vi "createTestCaseXMLReport.vi"(8 "error in (no error)":errorcluster, 11 "TestTestResult.Ant":refnum<class "_TextTestResult.JUnitXML.lvclass">) -> (0 "error out":errorcluster={"status"=TRUE, "code"=1, "source"="Release Queue in _TextTestResult.Ant.lvclass:createTestCaseXMLReport.vi"}, 2 "XML Report Data":string="<testsuite disabled=\"0\" errors=\"0\" failures=\"1\" name=\"TestSuite\" tests=\"1\" time=\"3405919291.7997\"><testsuite disabled=\"0\" errors=\"0\" failures=\"2\" name=\"MixedTest TestSuite\" tests=\"3\" time=\"3405919291.7997\"><testsuite disabled=\"0\" errors=\"0\" failures=\"1\" name=\"FrameworkSubTestSuite\" tests=\"2\" time=\"1.3519439697266\"><testcase classname=\"DoNotWaitOnTestComplete\" name=\"testDemo2\" status=\"testPass\" time=\"0.010014533996582\"/><testcase classname=\"DoNotWaitOnTestComplete\" name=\"testDemo\" status=\"testFailure\" time=\"0.010014533996582\"/></TestSuite><testsuite disabled=\"0\" errors=\"0\" failures=\"2\" name=\"FrameworkSubTestSuite\" tests=\"2\" time=\"1.6123185157776\"><testcase classname=\"DoNotWaitOnTestComplete\" name=\"testDemo2\" status=\"testPass\" time=\"0.010014057159424\"/><testcase classname=\"DoNotWaitOnTestComplete\" name=\"testDemo\" status=\"testFailure\" time=\"0.010014057159424\"/><testcase classname=\"LocationOutsideClassRoot\" name=\"testOutsideRoot\" status=\"testFailure\" time=\"0.010014533996582\"/>")   [LabVIEW 2018, in "_TextTestResult.JUnitXML.lvclass"]
uses:
  _TextTestResult.JUnitXML.lvclass
  _TextTestResult.JUnitXML.lvclass/_TextTestResult.JUnitXML.ctl
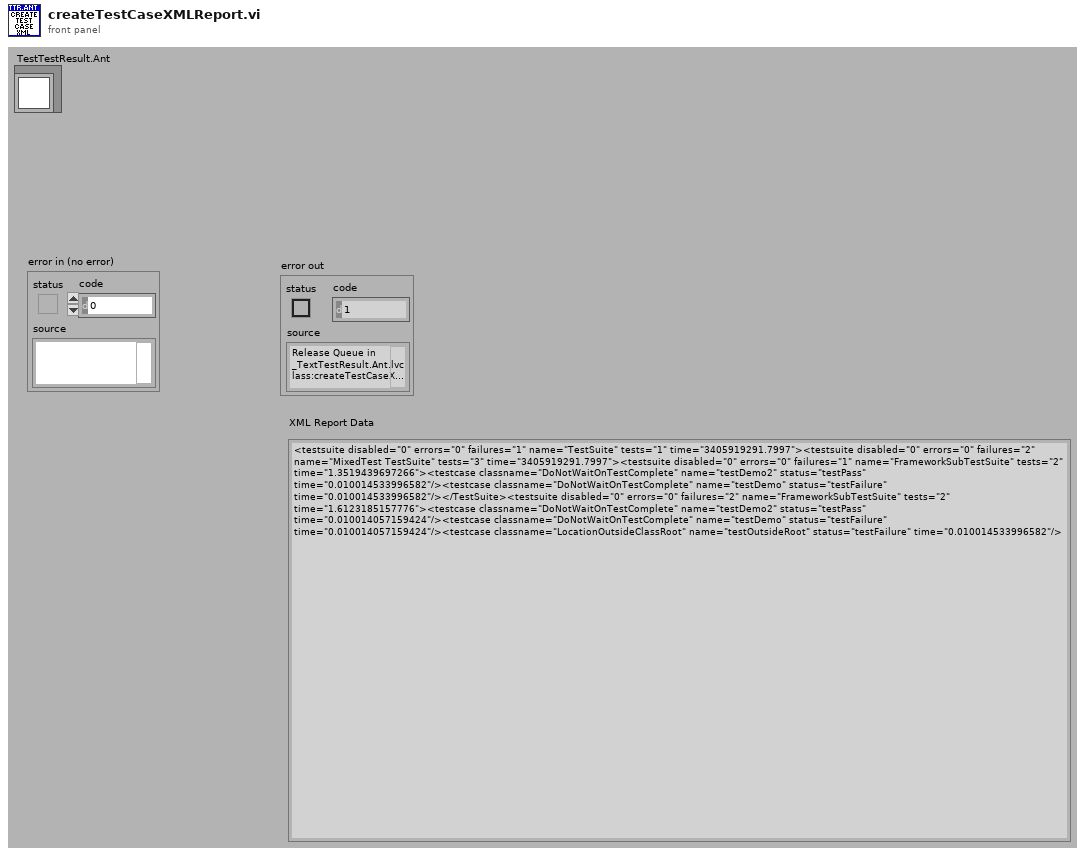
[diagram p1: front panel]
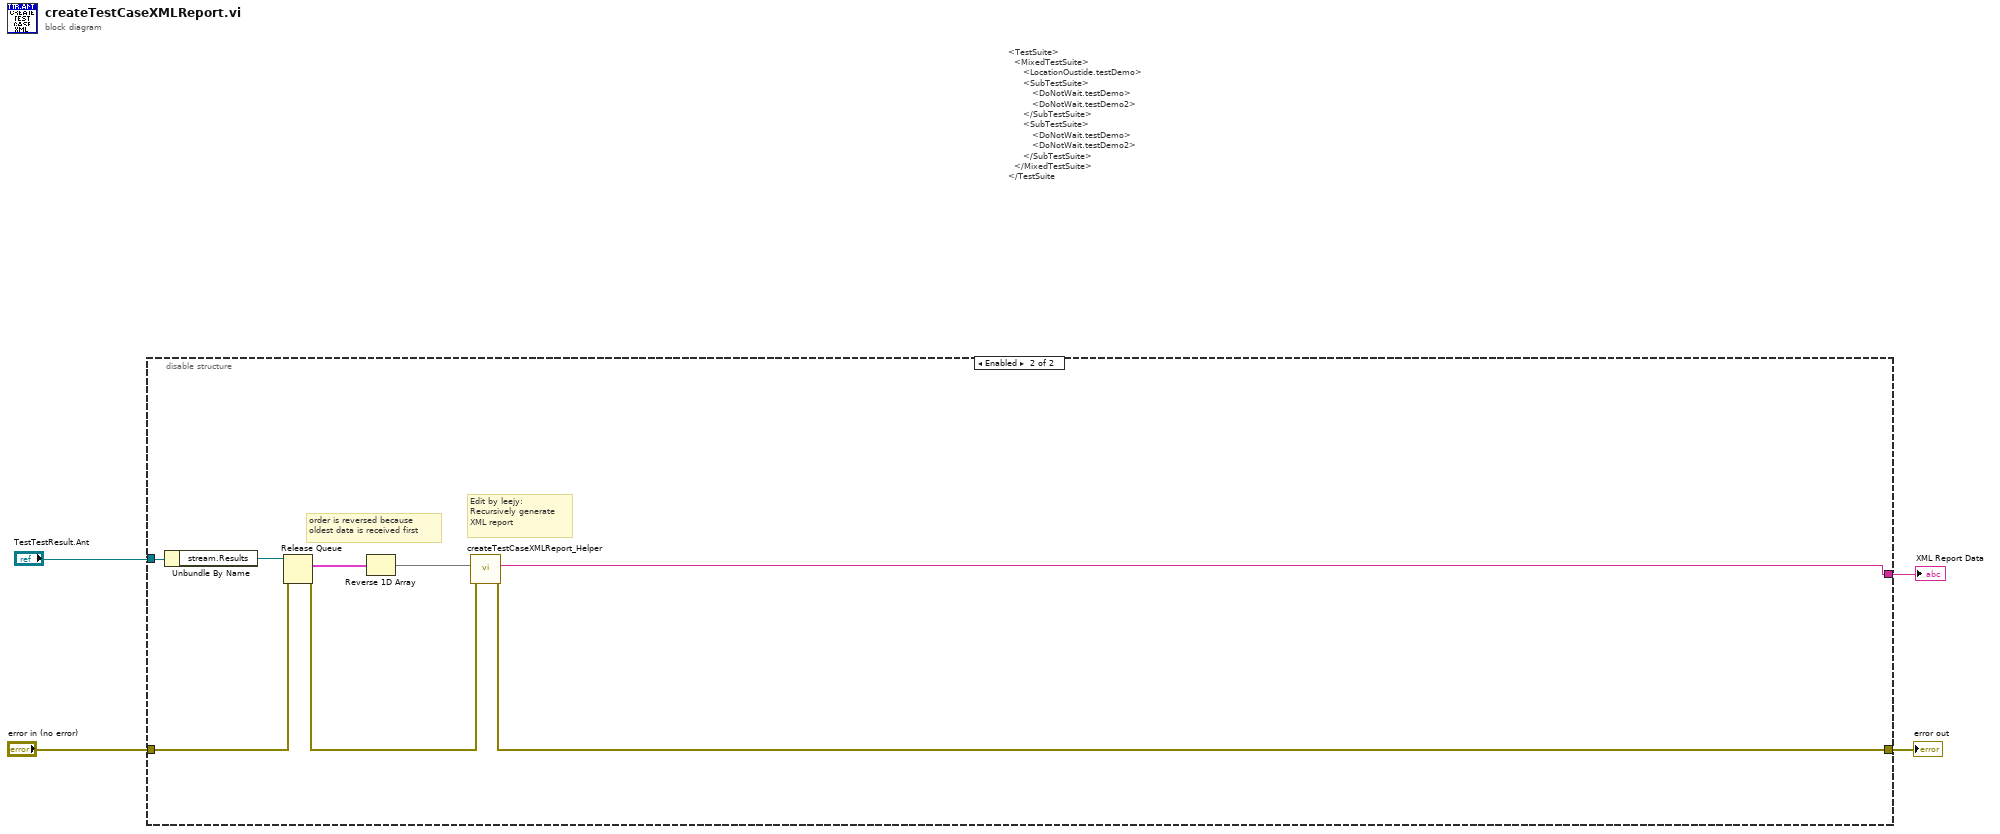
[diagram p0: block diagram]
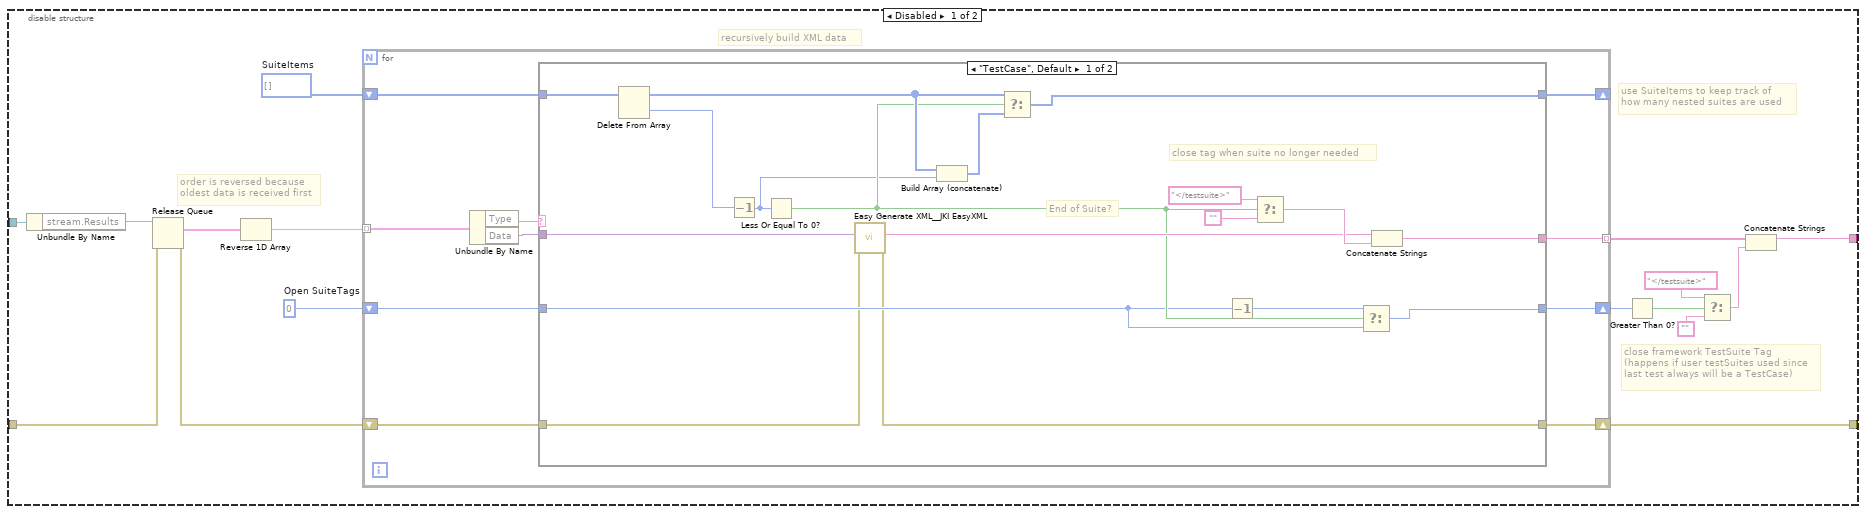
[diagram p2: hidden frame]
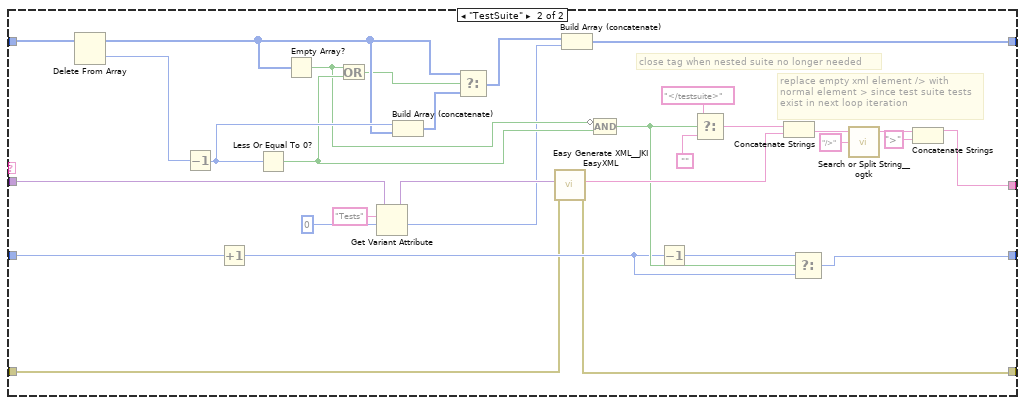
[diagram p3: hidden frame]
diagram:
  # "<TestSuite>\n  <MixedTestSuite>\n     <LocationOustide.testDemo>\n     <SubTestSuite>\n        <DoNotWait.testDemo>\n        <DoNotWait.testDemo2>\n     </SubTestSuite>\n     <SubTestSuite>\n        <DoNotWait.testDemo>\n        <DoNotWait.testDemo2>\n     </SubTestSuite>\n  </MixedTestSuite>\n</TestSuite"
  n1 = disable-structure shown="Enabled" {
    disable-tunnel: "TestTestResult.Ant" -> [w20 w85]
    disable-tunnel: "error in (no error)" -> [w18 w81]
    disable-tunnel: [w14 w82] -> w2
    disable-tunnel: [w5 w83] -> w1
    frame Disabled {
      w12 = 0  # Open SuiteTags
      w17 = i32[] []  # SuiteItems
      # "close framework TestSuite Tag\n(happens if user testSuites used since\nlast test always will be a TestCase)"
      # "recursively build XML data"
      # "use SuiteItems to keep track of\nhow many nested suites are used"
      # "order is reversed because\noldest data is received first"
      n2 = Unbundle By Name(w20) -> ("stream.Results"=w19:refnum<queue>)
      n3 = Release Queue(queue=w19, error in (no error)=w18) -> (remaining elements=w16:cluster{"Type":string, "Data":variant}[], error out=w6:errorcluster)  [unwired: 1 in, 1 out]
      n4 = Reverse 1D Array(array=w16) -> (reversed array=w13:cluster{"Type":string, "Data":variant}[])
      n5 = for {
        tunnel: [w28] -> w15 mode=indexing
        shift-right: [w26] -> _
        shift-left: w17 -> [w27]
        tunnel: w13 -> [w25] mode=indexing
        shift-right: [w23] -> w11
        shift-left: w12 -> [w24]
        shift-right: [w21] -> w5
        shift-left: w6 -> [w22]
        n6 = Unbundle By Name(w25) -> ("Type"=w30:string, "Data"=w29:variant)
        n7 = case shown="\"TestCase\", Default" w30 {
          tunnel: w29 -> [w48 w54]
          tunnel: [w47 w61] -> w28
          tunnel: w27 -> [w43 w71]
          tunnel: [w33 w68] -> w26
          tunnel: w24 -> [w38 w60]
          tunnel: [w37 w56] -> w23
          tunnel: w22 -> [w32 w50]
          tunnel: [w31 w49] -> w21
          frame "TestCase", Default {
            # "close tag when suite no longer needed"
            # "End of Suite?"
            n8 = Delete From Array(array=w43) -> (deleted portion=w46:i32, array with subset deleted=w44:i32[])  [unwired: 2 in]
            n9 = Decrement(x=w46) -> (x-1=w34:i32)
            n10 = Less Or Equal To 0?(x=w34) -> (x <= 0?=w39:bool)
            n11 = call <vilib>:"Easy Generate XML__JKI EasyXML.vi"("error in (no error)"=w32, "LabVIEW Data"=w48) -> ("error out"=w31:errorcluster, "XML String"=w41:string)  [unwired: 8 in]
            n12 = Build Array (concatenate)(w44, w34) -> (w45:i32[])
            n13 = Select(t=w44, s=w39, f=w45) -> (s? t:f=w33:i32[])
            n14 = Decrement(x=w38) -> (x-1=w40:i32)
            n15 = Select(t="</testsuite>" ("string"), s=w39, f="") -> (s? t:f=w42:string)
            n16 = Select(t=w40, s=w39, f=w38) -> (s? t:f=w37:i32)
            n17 = Concatenate Strings(w41, w42) -> (w47:string)
          }
          frame "TestSuite" {
            # "replace empty xml element /> with\nnormal element > since test suite tests\nexist in next loop iteration"
            # "close tag when nested suite no longer needed"
            n18 = Delete From Array(array=w71) -> (deleted portion=w76:i32, array with subset deleted=w70:i32[])  [unwired: 2 in]
            n19 = Decrement(x=w76) -> (x-1=w73:i32)
            n20 = Increment(x=w60) -> (x+1=w57:i32)
            n21 = Less Or Equal To 0?(x=w73) -> (x <= 0?=w66:bool)
            n22 = Empty Array?(array=w70) -> (empty?=w65:bool)
            n23 = Or(x=w65, y=w66) -> (x .or. y?=w67:bool)
            n24 = Get Variant Attribute(Variant=w54, name="Tests", default value (empty Variant)=0 ("size(s)")) -> (duplicate Variant=w53:variant, value=w51:i32)  [unwired: 1 in, 2 out]
            n25 = Build Array (concatenate)(w73, w70) -> (w72:i32[])
            n26 = Select(t=w70, s=w67, f=w72) -> (s? t:f=w69:i32[])
            n27 = call <vilib>:"Easy Generate XML__JKI EasyXML.vi"("error in (no error)"=w50, "LabVIEW Data"=w53) -> ("error out"=w49:errorcluster, "XML String"=w63:string)  [unwired: 8 in]
            n28 = Build Array (concatenate)(w69, w51) -> (w68:i32[])
            n29 = Compound Arithmetic op=AND(invert w65, w66) -> (w58:bool)
            n30 = Decrement(x=w57) -> (x-1=w59:i32)
            n31 = Select(t="</testsuite>" ("string"), s=w58, f="") -> (s? t:f=w64:string)
            n32 = Concatenate Strings(w64, w63) -> (w62:string)
            n33 = Select(t=w59, s=w58, f=w57) -> (s? t:f=w56:i32)
            n34 = call <userlib>:"Search or Split String__ogtk.vi"("search string/char (-)"="/>", "string"=w62) -> ("substring before match"=w78:string)  [unwired: 1 in, 2 out]
            n35 = Concatenate Strings(w78, ">" ("string")) -> (w61:string)
          }
        }
      }
      n36 = Greater Than 0?(x=w11) -> (x > 0?=w10:bool)
      n37 = Select(t="</testsuite>" ("string"), s=w10, f="") -> (s? t:f=w7:string)
      n38 = Concatenate Strings(w15, w7) -> (w14:string)
    }
    frame Enabled {
      # "Edit by leejy:\nRecursively generate\nXML report"
      # "order is reversed because\noldest data is received first"
      n39 = Unbundle By Name(w85) -> ("stream.Results"=w87:refnum<queue>)
      n40 = Release Queue(queue=w87, error in (no error)=w81) -> (remaining elements=w86:cluster{"Type":string, "Data":variant}[], error out=w80:errorcluster)  [unwired: 1 in, 1 out]
      n41 = Reverse 1D Array(array=w86) -> (reversed array=w84:cluster{"Type":string, "Data":variant}[])
      n42 = call "createTestCaseXMLReport_Helper.vi"("error in (no error)"=w80, "remaining elements (internal - do not use)"=w84) -> ("error out"=w83:errorcluster, "XML string"=w82:string)  [unwired: 8 in]
    }
  }
  "error out" <- w1
  "XML Report Data" <- w2
